vi "check JSON validity.vi"(8 "error in (no error)":errorcluster, 11 "JSON string in":string="{\"status\":false,\"source\":\"\",\"code\":0,\"longdescr\":\"this is a looong description\"}") -> (0 "error out":errorcluster, 3 "JSON string out":string="{\"status\":false,\"source\":\"\",\"code\":0,\"longdescr\":\"this is a looong description\"}")   [LabVIEW 2018, in "LabView-0mq-Jl_Roundtrip_lib.lvlib"]
uses:
  LabView-0mq-Jl_Roundtrip_lib.lvlib
panel:
  out "unused value":i32
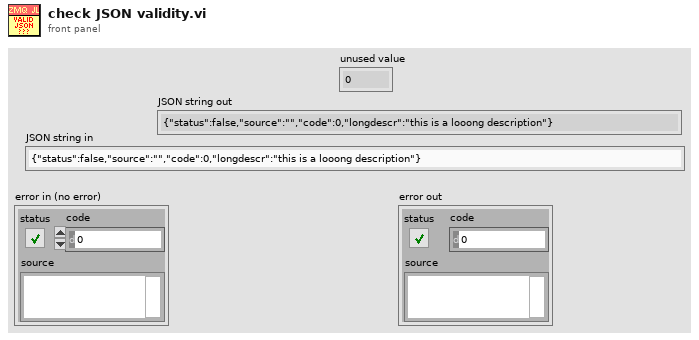
[diagram p1: front panel]
types:
  T1 = cluster{"unique_abracadabra_lfdhsdgihoggnksdihasd":i32}
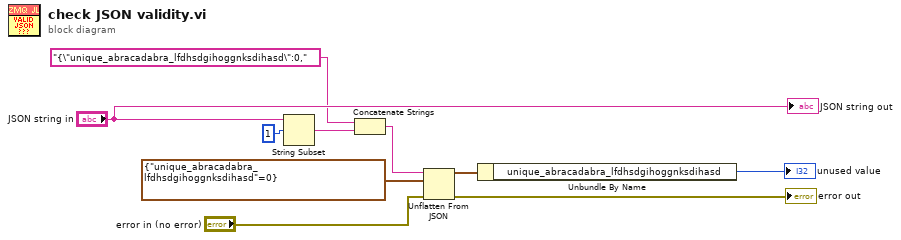
[diagram p0: block diagram]
diagram:
  n1 = String Subset(string="JSON string in", offset (0)=1) -> (substring=w4:string)  [unwired: 1 in]
  n2 = Concatenate Strings("{\"unique_abracadabra_lfdhsdgihoggnksdihasd\":0,", w4) -> (w2:string)
  n3 = Unflatten From JSON(JSON string=w2, type and defaults=T1 {"unique_abracadabra_lfdhsdgihoggnksdihasd"=0}, error in (no error)="error in (no error)") -> (value=w10:T1, error out=→"error out":errorcluster)  [unwired: 4 in]
  n4 = Unbundle By Name(w10) -> ("unique_abracadabra_lfdhsdgihoggnksdihasd"=→"unused value":i32)
  "JSON string out" <- "JSON string in"
